vi "GUID2.vi"() -> (3 "trimmed string":string caption="GUID")   [LabVIEW 2020]
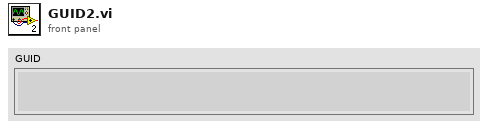
[diagram p1: front panel]
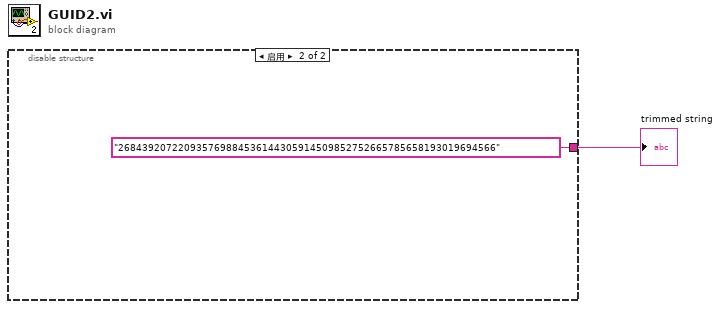
[diagram p0: block diagram]
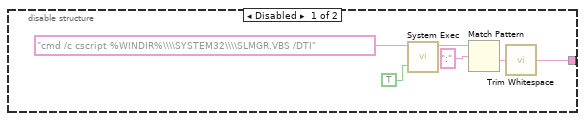
[diagram p2: hidden frame]
diagram:
  n1 = disable-structure shown="启用" {
    disable-tunnel: [w2 "268439207220935769884536144305914509852752665785658193019694566" ("trimmed string")] -> w1
    frame Disabled {
      n2 = call <vilib>:"System Exec.vi"("run minimized? (F)"=TRUE, "command line"="cmd /c cscript %WINDIR%\\\\SYSTEM32\\\\SLMGR.VBS /DTI") -> ("standard output"=w5:string)  [unwired: 6 in, 3 out]
      n3 = Match Pattern(string=w5, regular expression=":" ("正则表达式")) -> (after substring=w3:string)  [unwired: 1 in, 3 out]
      n4 = call <vilib>:"Trim Whitespace.vi"("string"=w3) -> ("trimmed string"=w2:string)  [unwired: 1 in]
    }
    frame Enabled {
    }
  }
  "trimmed string" <- w1
